vi "Tesla_Test_v3.vi"() -> ()   [LabVIEW 2013]
uses:
  General VIs/Tesla/Control/Command Enum.ctl
  <vilib>/Utility/NIReport.llb/NI_report.lvclass
  <vilib>/Utility/NIReport.llb/Append Report Text (str wrap).vi
  <vilib>/regexp/Match Regular Expression.xnode
panel:
  out "index":i32
  in  "error in":errorcluster
  out "error out":errorcluster
  in  "Tab Control":T1(tab)
  in  "Protocol":bool
  in  "Text Base":bool
  in  "Network":bool
  in  "Commence":bool
  out "IP address":i32
  out "offset past match":i32
  out "concatenated string":string
  out "Ping Cout":i32
  in  "file path":path=path "C:/Users/barddya/Desktop/Tesla/List_of_IPs.txt"
  out "VP/F1 5":bool
  out "VP/F1 4":bool
  out "VP/F1 3":bool
  out "VP/F1 2":bool
  out "VP/F1":bool
  out "Hex 5":bool
  out "Hex 4":bool
  out "Hex 3":bool
  out "Hex 2":bool
  out "Hex 1":bool
  out "Percent 5":dbl
  out "Percent 4":dbl
  out "Percent 3":dbl
  out "Percent 2":dbl
  out "Percent 1":dbl
  out "Voltage 5":dbl
  out "Voltage 4":dbl
  out "Voltage 3":dbl
  out "Voltage 2":dbl
  out "Voltage 1":dbl
  out "Pass/Fail1 5":bool
  out "Pass/Fail1 4":bool
  out "Pass/Fail1 3":bool
  out "Pass/Fail1 2":bool
  out "Pass/Fail1":bool
  in  "Path to Text Base Comm":path=path "C:/Users/barddya/Desktop/Tesla/test2.txt"
  out "Value in Flpating Point":dbl
  out "Hex String":string
  in  "Path Protocol test":path=path "C:/Users/barddya/Desktop/Tesla_Program/test3.bin"
  in  "Panic Stop Stop":bool=TRUE
  in  "Done press continue":bool
  # "Pass/Fail"
  # "Voltage"
  # "Precent"
  # "Is Hex"
  # "Results"
  # "Response 1"
  # "Response 2"
  # "Response 3"
  # "Response 4"
  # "Response 5"
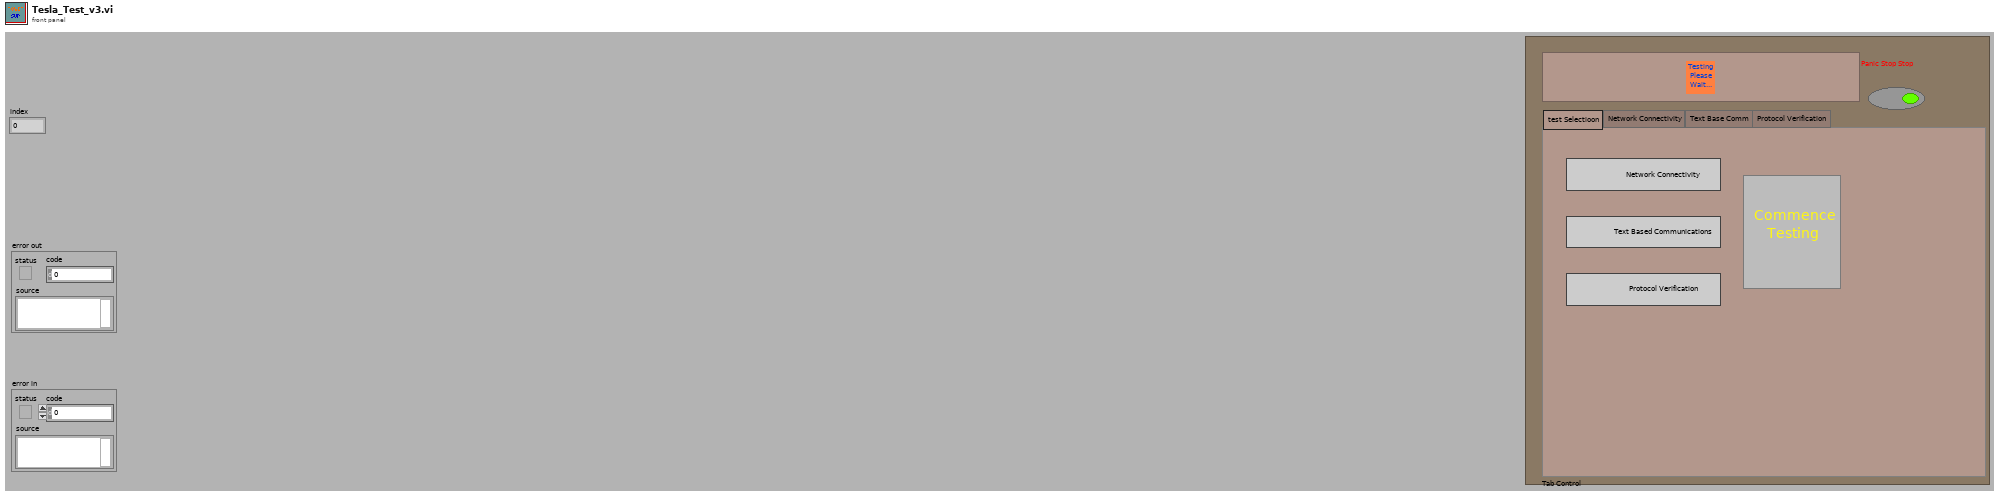
[diagram p1: front panel]
types:
  T1 = enum32{"test Selectioon", "Network Connectivity", "Text Base Comm", "Protocol Verification"}
  T2 = typedef "Command Enum.ctl" = enum16{"Test Selection", "Network", "Text Base", "Protocol", "Restart_Print", "Stop"}
  T3 = enum16{"big-endian, network order", "native, host order", "little-endian"}
  T4 = enum16{"open", "replace", "create", "open or create", "replace or create", "replace or create with confirmation"}
  T5 = cluster{"Charset (-1)":i16, "Weight (-1)":i16, "Name":string, "Size":string}
  T6 = enum16{"Standard Report", "HTML", "Word", "Excel"}
  T7 = cluster{"output state":bool, "Device ID":i32, "Set CC current":dbl}
  T8 = enum16{"Left Button", "Center Button", "Right Button", "Window Close"}
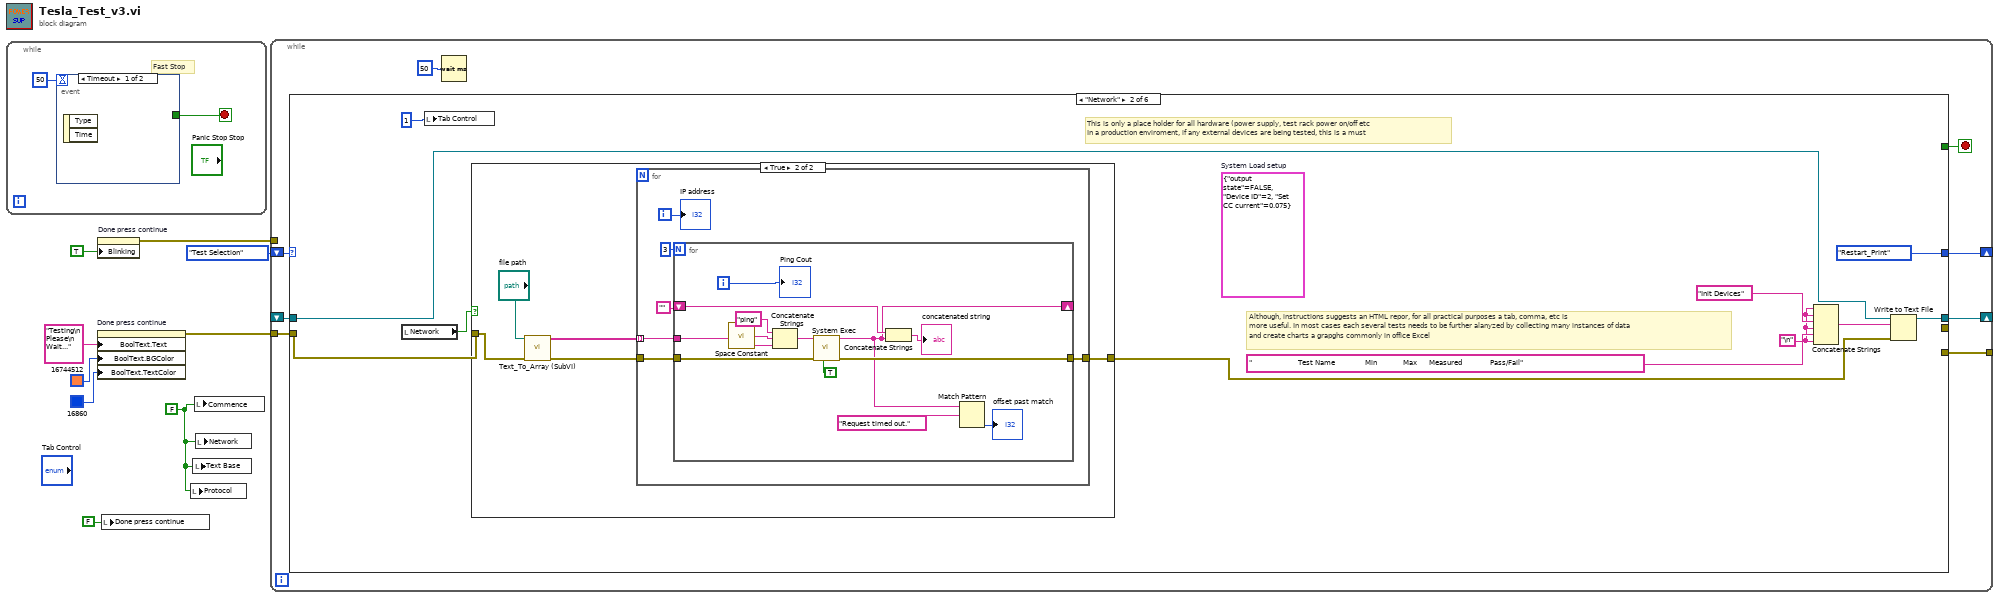
[diagram p0: block diagram]
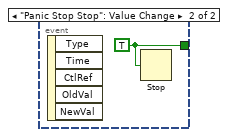
[diagram p2: hidden frame]
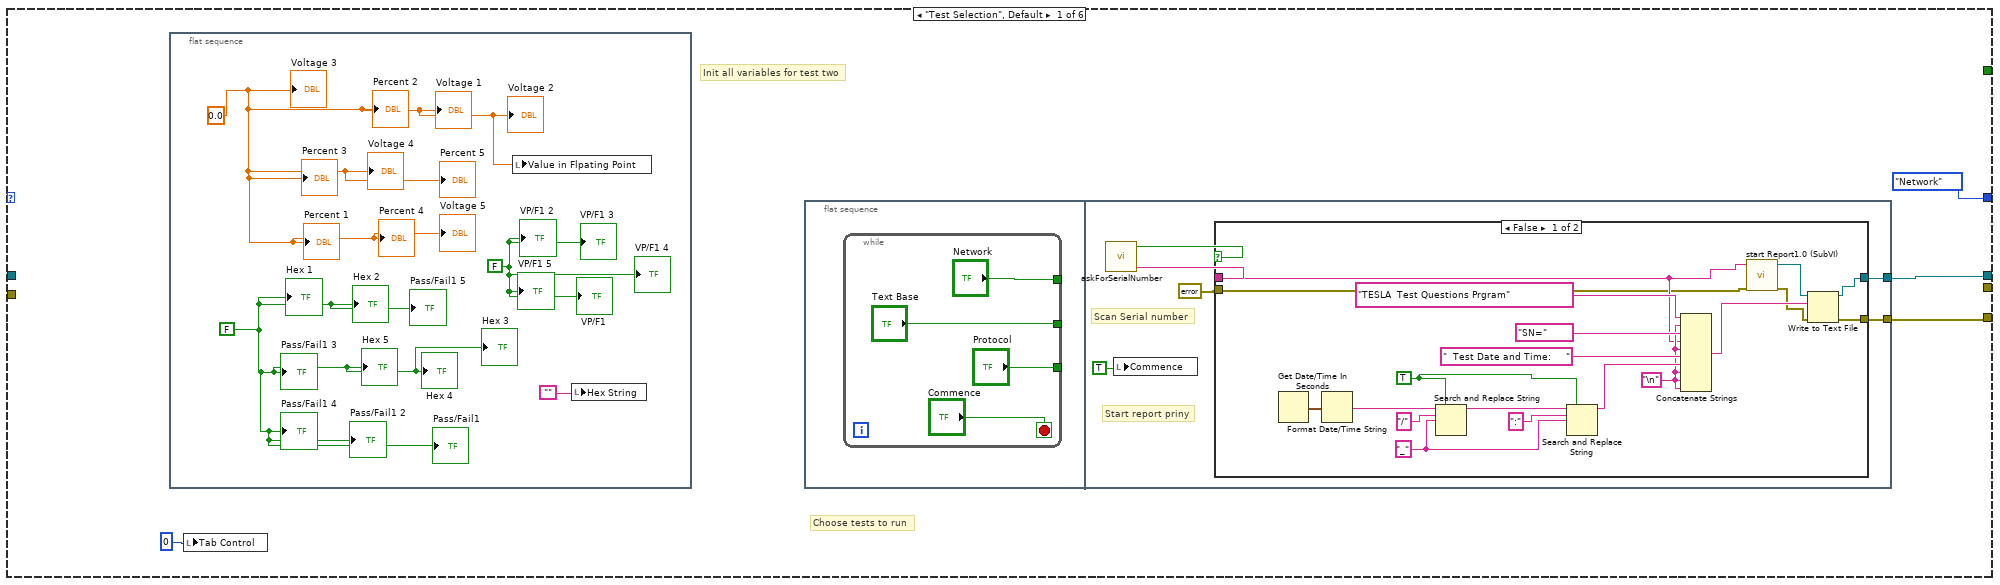
[diagram p3: hidden frame]
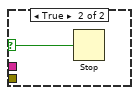
[diagram p4: hidden frame]
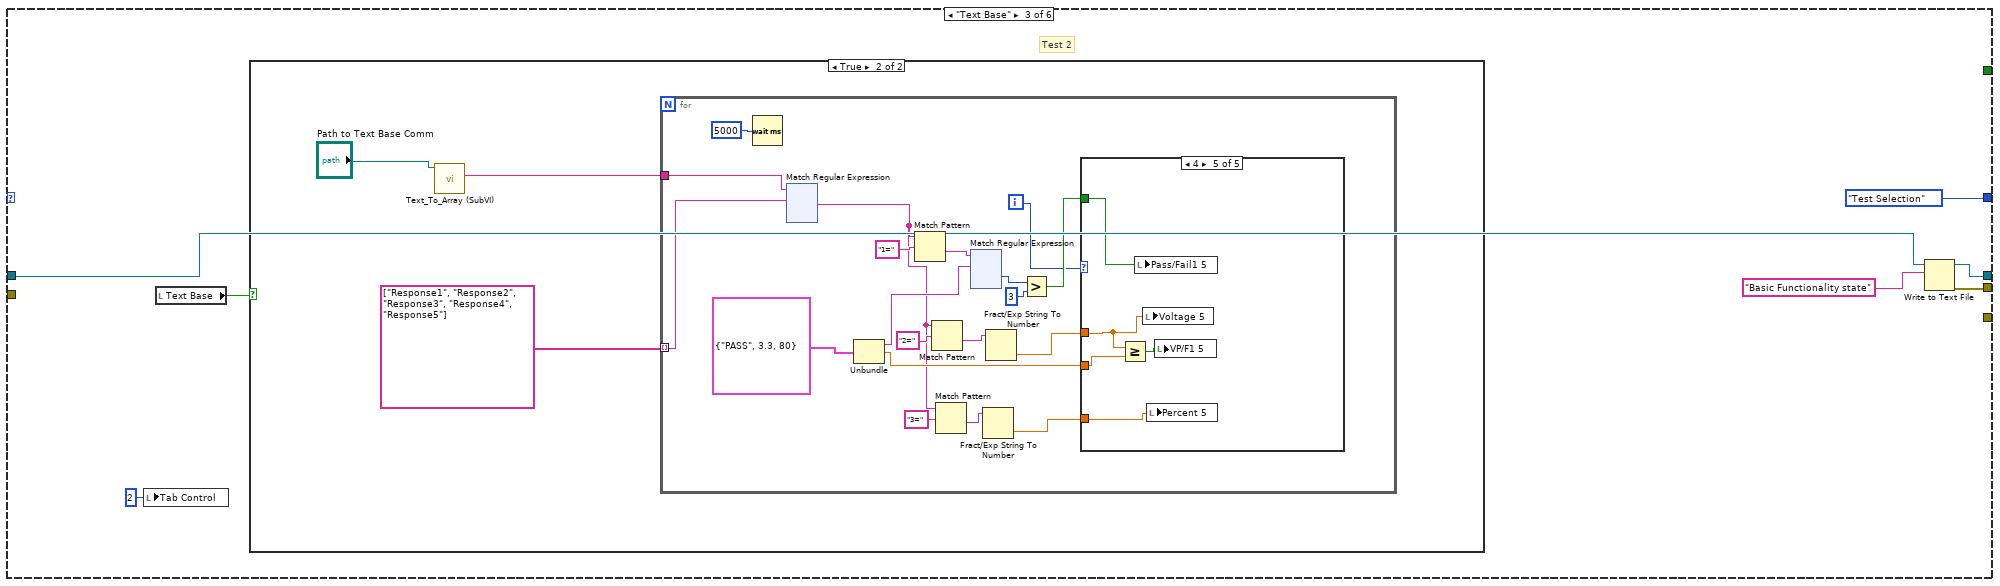
[diagram p6: hidden frame]
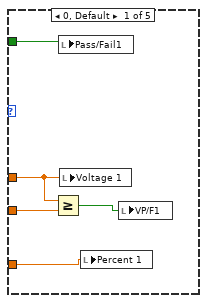
[diagram p8: hidden frame]
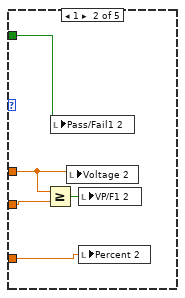
[diagram p9: hidden frame]
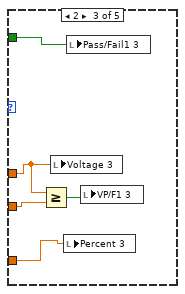
[diagram p10: hidden frame]
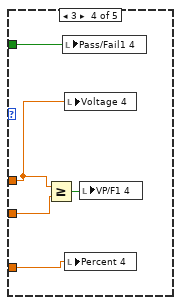
[diagram p11: hidden frame]
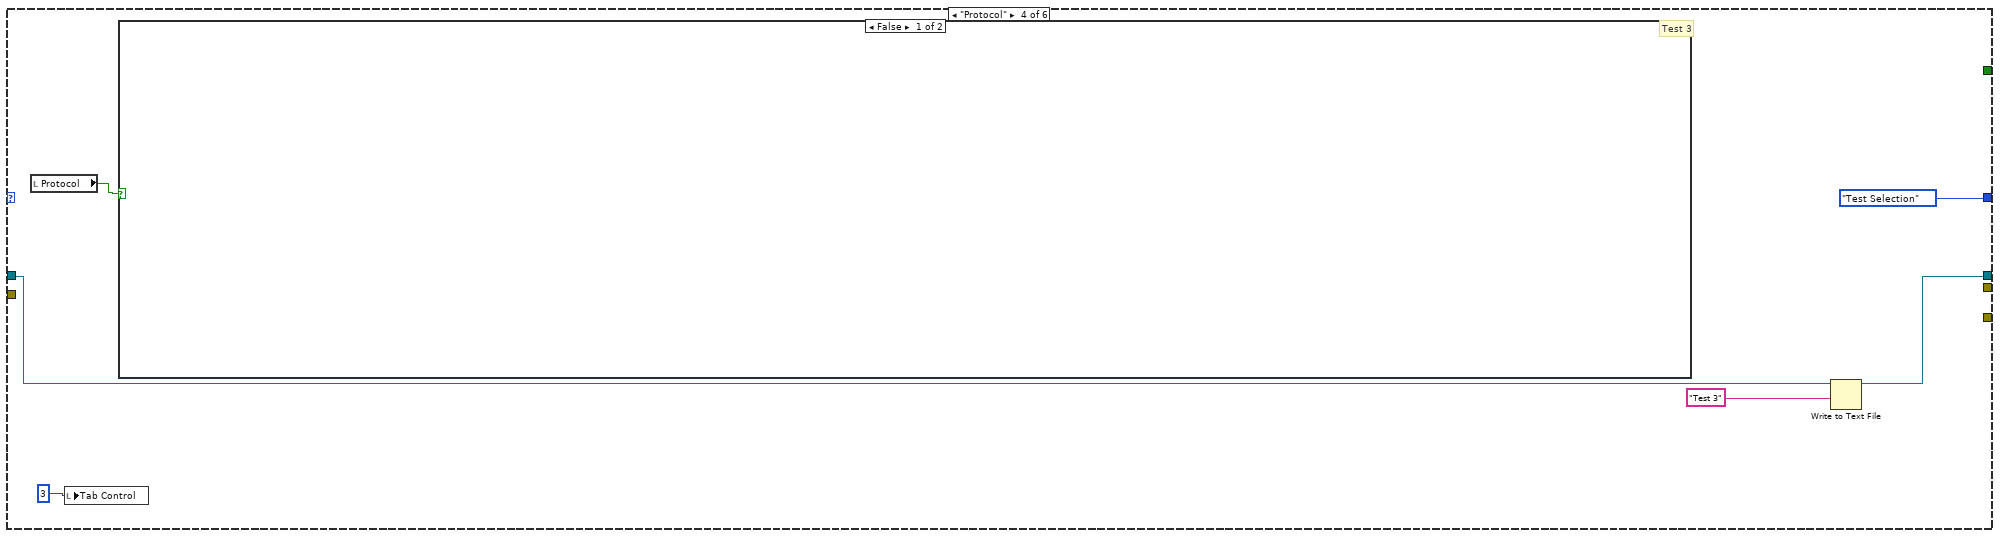
[diagram p12: hidden frame]
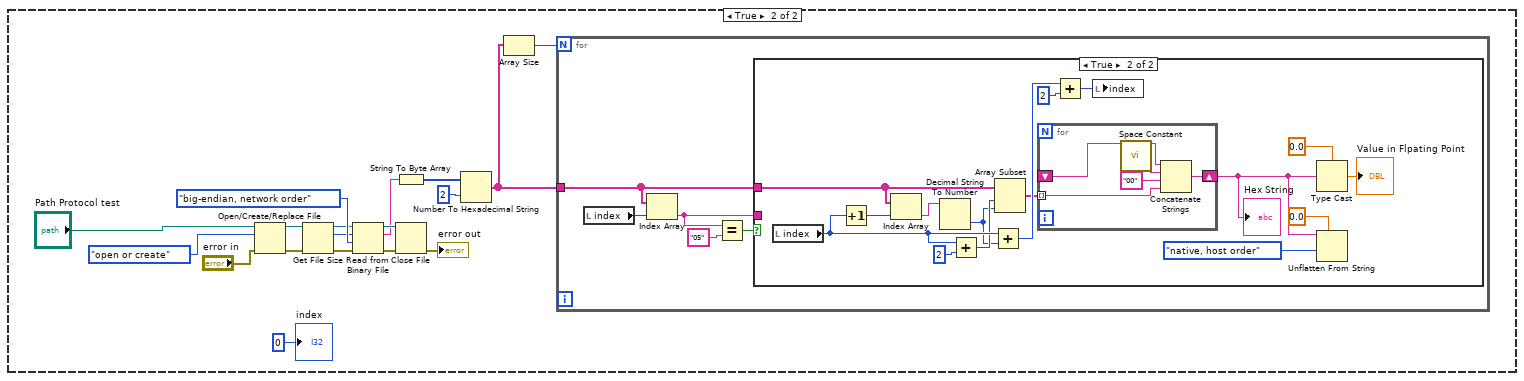
[diagram p13: hidden frame]
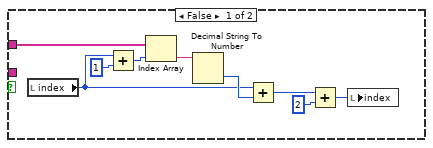
[diagram p14: hidden frame]
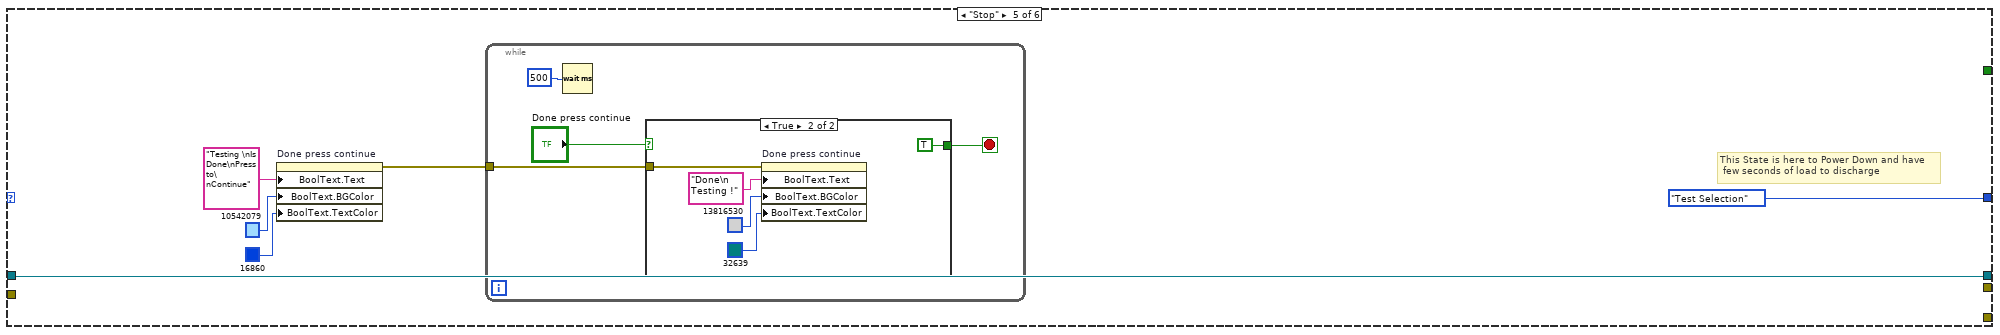
[diagram p15: hidden frame]
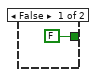
[diagram p16: hidden frame]
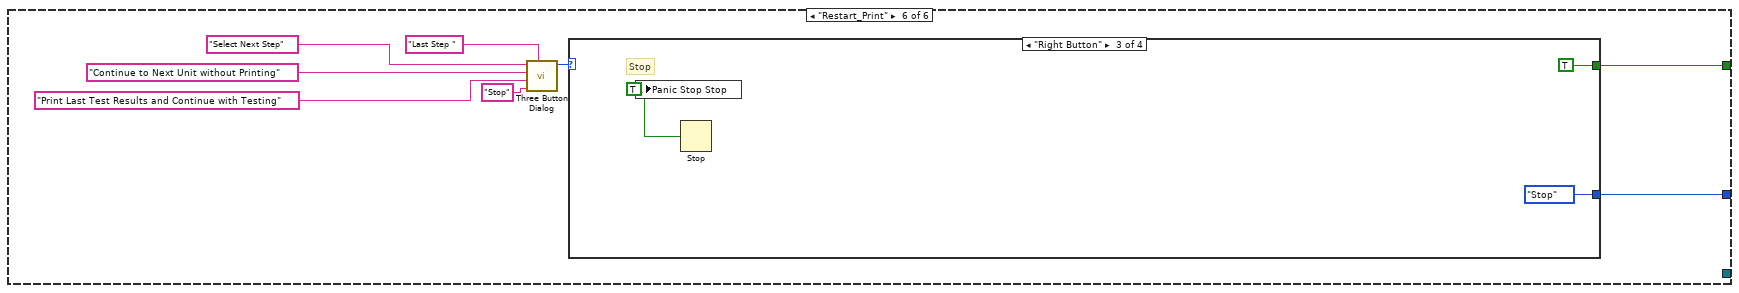
[diagram p17: hidden frame]
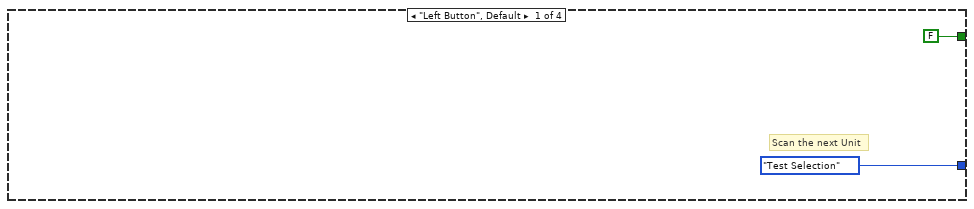
[diagram p18: hidden frame]
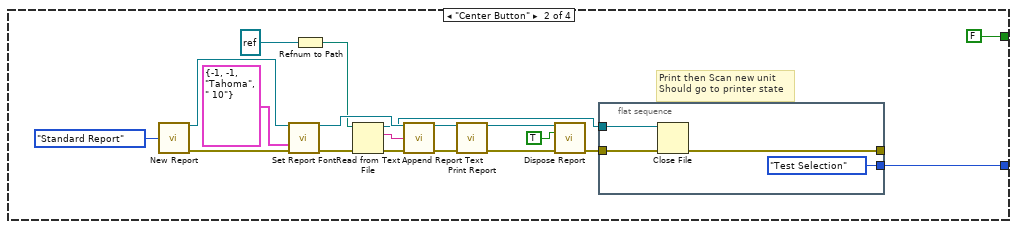
[diagram p19: hidden frame]
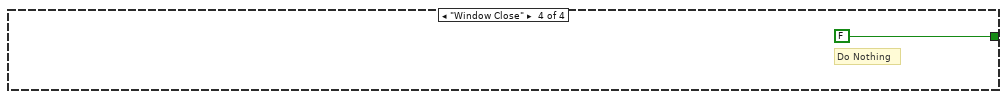
[diagram p20: hidden frame]
diagram:
  w1 = FALSE
  n1 = while {
    stop <- w10 stop-if-true
    # "Fast Stop"
    n2 = event shown="[0] Timeout" {
      selector: _ -> [_ _]
      dyn-events: _ -> [_ _]
      timeout: 50 -> [_ _]
      tunnel: [_ w12] -> w10
      event Timeout {
        n3 = event-data() -> ()  [unwired: 1 in, 2 out]
      }
      event "Panic Stop Stop": Value Change {
        w12 = TRUE
        n4 = event-data() -> ()  [unwired: 1 in, 5 out]
        n5 = Stop(stop? (T)=w12) -> ()
      }
    }
  }
  n6 = property on="Done press continue" class="Bool (strict)"("BoolText.Text"="Testing\n Please\n Wait...", "BoolText.BGColor"=u32 16744512, "BoolText.TextColor"=u32 16860) -> (error out=w7:errorcluster)  [unwired: 2 in, 1 out]
  n7 = property on="Done press continue" class="Bool (strict)"("Blinking"=TRUE) -> (error out=w3:errorcluster)  [unwired: 2 in, 1 out]
  n8 = local write "Done press continue"(FALSE) -> ()
  n9 = local write "Protocol"(w1) -> ()
  n10 = local write "Text Base"(w1) -> ()
  n11 = local write "Commence"(w1) -> ()
  n12 = local write "Network"(w1) -> ()
  n13 = while {
    shift-right: [w19] -> _
    shift-left: Command_Enum."Test Selection" ("Command Enum") -> [w20]
    tunnel: w7 -> [w16]
    tunnel: w3 -> [_]
    shift-right: [w15] -> _
    shift-left: _ -> [w14]
    tunnel: [w13] -> _
    stop <- w18 stop-if-true
    n14 = case shown="\"Network\"" w20 {
      tunnel: [Command_Enum."Network" ("Command Enum") Command_Enum."Restart_Print" ("Command Enum") Command_Enum."Test Selection" ("Command Enum") Command_Enum."Test Selection" ("Command Enum") Command_Enum."Test Selection" ("Command Enum") w453] -> w19
      tunnel: [_ _ _ _ _ w452] -> w18
      tunnel: w16 -> [_ w62 _ _ _ _]
      tunnel: [w23 w67 w99 w381 w436 _] -> w15
      tunnel: w14 -> [_ w66 w98 w379 w436 _]
      tunnel: [_ _ w100 _ _ _] -> _
      tunnel: [w21 _ _ _ _ _] -> w13
      frame "Test Selection", Default {
        # "Choose tests to run"
        # "Init all variables for test two"
        n15 = flat-sequence {
          frame #0 {
            w27 = FALSE
            w28 = FALSE
            w26 = 0.0
            n16 = local write "Value in Flpating Point"(w26) -> ()
            n17 = local write "Hex String"("") -> ()
            "Voltage 5" <- w26
            "Percent 5" <- w26
            "Voltage 3" <- w26
            "Voltage 4" <- w26
            "Voltage 2" <- w26
            "Percent 4" <- w26
            "Percent 3" <- w26
            "Voltage 1" <- w26
            "Percent 2" <- w26
            "Percent 1" <- w26
            "Pass/Fail1 5" <- w28
            "Hex 5" <- w28
            "Pass/Fail1 3" <- w28
            "Pass/Fail1 4" <- w28
            "Pass/Fail1" <- w28
            "Hex 3" <- w28
            "Hex 4" <- w28
            "Hex 2" <- w28
            "Hex 1" <- w28
            "Pass/Fail1 2" <- w28
            "VP/F1 3" <- w27
            "VP/F1 4" <- w27
            "VP/F1 2" <- w27
            "VP/F1" <- w27
            "VP/F1 5" <- w27
          }
        }
        n18 = local write "Tab Control"(0) -> ()
        n19 = flat-sequence {
          tunnel: [w36] -> w23
          tunnel: [w35] -> w21
          frame #0 {
            n20 = while {
              tunnel: ["Network"] -> _
              tunnel: ["Text Base"] -> _
              tunnel: ["Protocol"] -> _
              stop <- "Commence" stop-if-true
            }
          }
          frame #1 {
            # "Start report priny"
            # "Scan Serial number"
            n21 = call "askForSerialNumber.vi"() -> ("Stop"=w38:bool, "Serial Number scanned"=w37:string)  [unwired: 1 in, 1 out]
            n22 = local write "Commence"(TRUE) -> ()
            n23 = case shown="False" w38 {
              selector: w38 -> [_ w58]
              tunnel: w37 -> [w42 _]
              tunnel: [w45 _] -> w36
              tunnel: [w43 _] -> w35
              tunnel: errorcluster {"status"=FALSE, "code"=0, "source"=""} ("error constant") -> [w41 _]
              frame False {
                w46 = "\n"
                w55 = TRUE ("replace all? (F)")
                w54 = "_"
                n24 = Get Date/Time In Seconds() -> (seconds since 1Jan1904=w49:timestamp)
                n25 = Format Date/Time String(seconds (now)=w49) -> (date/time string=w50:string)  [unwired: 2 in]
                n26 = Search and Replace String(replace all?=w55, input string=w50, search string="/", replace string=w54) -> (result string=w52:string)  [unwired: 4 in, 3 out]
                n27 = Search and Replace String(replace all?=w55, input string=w52, search string=":", replace string=w54) -> (result string=w57:string)  [unwired: 4 in, 3 out]
                n28 = Concatenate Strings("TESLA  Test Questions Prgram", w46, "SN=", w42, w46, "  Test Date and Time:     ", w57, w46, w46, w46) -> (w44:string)
                n29 = call "start Report1.0 (SubVI).vi"("error in (no error)"=w41, "Serial Number"=w42) -> ("error out"=w40:errorcluster, "Byte Stream File out"=w39:refnum<file>)  [unwired: 8 in]
                n30 = Write to Text File(file (use dialog)=w39, text=w44, error in=w40) -> (refnum out=w45:refnum<file>, error out=w43:errorcluster)  [unwired: 1 in, 1 out]
              }
              frame True {
                n31 = Stop(stop? (T)=w58) -> ()
              }
            }
          }
        }
      }
      frame "Network" {
        w63 = "\n"
        (unwired) T7 {"output state"=FALSE, "Device ID"=2, "Set CC current"=0.075}  # System Load setup
        # "Although, instructions suggests an HTML repor, for all practical purposes a tab, comma, etc is \nmore useful. In most cases each several tests needs to be further alanyzed by collecting many instances of data \nand create charts a grapghs commonly in office Excel"
        # "This is only a place holder for all hardware (power supply, test rack power on/off etc\nIn a production enviroment, if any external devices are being tested, this is a must"
        n32 = local read "Network"() -> (w59:bool)
        n33 = local write "Tab Control"(1) -> ()
        n34 = case shown="True" w59 {
          tunnel: w62 -> [w70 w72]
          tunnel: [w70 w71] -> w61
          frame False {
          }
          frame True {
            n35 = call "Text_To_Array (SubVI).vi"("error in (no error)"=w72, "file path"="file path") -> ("error out"=w74:errorcluster, "Array"=w75:string[])  [unwired: 7 in, 1 out]
            n36 = for {
              tunnel: w75 -> [w79] mode=indexing
              tunnel: w74 -> [w81]
              tunnel: [w80] -> w71
              i -> [w77]
              n37 = for {
                N: 3 -> [_]
                tunnel: w81 -> [w94]
                tunnel: [w93] -> w80
                tunnel: w79 -> [w91]
                shift-right: [w84] -> _
                shift-left: "" -> [w86]
                i -> [w87]
                n38 = call <vilib>:"Space Constant.vi"() -> ("String"=w89:string)
                n39 = Concatenate Strings("ping", w89, w91) -> (w92:string)
                n40 = call <vilib>:"System Exec.vi"("run minimized? (F)"=TRUE, "error in (no error)"=w94, "command line"=w92) -> ("error out"=w93:errorcluster, "standard output"=w84:string)  [unwired: 5 in, 2 out]
                n41 = Concatenate Strings(w86, w84) -> (→"concatenated string":string)
                n42 = Match Pattern(string=w84, regular expression="Request timed out." ("search string/char (-)")) -> (offset past match=→"offset past match":i32)  [unwired: 1 in, 3 out]
                "Ping Cout" <- w87
              }
              "IP address" <- w77
            }
          }
        }
        n43 = Concatenate Strings(w63, w63, "Init Devices", w63, "                       Test Name               Min             Max      Measured              Pass/Fail", w63) -> (w68:string)
        n44 = Write to Text File(file (use dialog)=w66, text=w68, error in=w61) -> (refnum out=w67:refnum<file>)  [unwired: 1 in, 2 out]
      }
      frame "Text Base" {
        # "Test 2"
        n45 = local write "Tab Control"(2) -> ()
        n46 = local read "Text Base"() -> (w96:bool)
        n47 = case shown="True" w96 {
          frame False {
          }
          frame True {
            n48 = call "Text_To_Array (SubVI).vi"("file path"="Path to Text Base Comm") -> ("text"=w103:string)  [unwired: 8 in, 2 out]
            n49 = for {
              tunnel: w103 -> [w112]
              tunnel: string[] ["Response1", "Response2", "Response3", "Response4", "Response5"] -> [w111] mode=indexing
              i -> [w110]
              n50 = Wait (ms)(milliseconds to wait=5000) -> ()  [unwired: 1 out]
              n51 = xnode "Match Regular Expression"("input string"=w112, "regular expression"=w111) -> ("after match"=w107:string)  [unwired: 4 in, 4 out]
              n52 = Unbundle(cluster{string, dbl, i32} {"PASS", 3.3, 80}) -> (w122:string, w109:dbl)  [unwired: 1 out]
              n53 = Match Pattern(string=w107, regular expression="1=") -> (after substring=w119:string)  [unwired: 1 in, 3 out]
              n54 = Match Pattern(string=w107, regular expression="2=") -> (after substring=w114:string)  [unwired: 1 in, 3 out]
              n55 = Match Pattern(string=w107, regular expression="3=") -> (after substring=w106:string)  [unwired: 1 in, 3 out]
              n56 = xnode "Match Regular Expression"("input string"=w119, "regular expression"=w122) -> ("offset past match"=w118:i32)  [unwired: 4 in, 4 out]
              n57 = Fract/Exp String To Number(string=w106) -> (number=w105:dbl)  [unwired: 3 in, 1 out]
              n58 = Fract/Exp String To Number(string=w114) -> (number=w113:dbl)  [unwired: 3 in, 1 out]
              n59 = Greater?(x=w118, y=3) -> (0:w116:bool)
              n60 = case shown="4" w110 {
                tunnel: w116 -> [w128 w133 w138 w143 w148]
                tunnel: w113 -> [w127 w132 w137 w142 w147]
                tunnel: w109 -> [w126 w131 w136 w141 w146]
                tunnel: w105 -> [w124 w129 w134 w139 w144]
                frame 0, Default {
                  n61 = Greater Or Equal?(x=w127, y=w126) -> (x >= y?=w125:bool)
                  n62 = local write "Pass/Fail1"(w128) -> ()
                  n63 = local write "Voltage 1"(w127) -> ()
                  n64 = local write "Percent 1"(w124) -> ()
                  n65 = local write "VP/F1"(w125) -> ()
                }
                frame 1 {
                  n66 = Greater Or Equal?(x=w132, y=w131) -> (x >= y?=w130:bool)
                  n67 = local write "Pass/Fail1 2"(w133) -> ()
                  n68 = local write "Voltage 2"(w132) -> ()
                  n69 = local write "VP/F1 2"(w130) -> ()
                  n70 = local write "Percent 2"(w129) -> ()
                }
                frame 2 {
                  n71 = Greater Or Equal?(x=w137, y=w136) -> (x >= y?=w135:bool)
                  n72 = local write "Voltage 3"(w137) -> ()
                  n73 = local write "Percent 3"(w134) -> ()
                  n74 = local write "Pass/Fail1 3"(w138) -> ()
                  n75 = local write "VP/F1 3"(w135) -> ()
                }
                frame 3 {
                  n76 = Greater Or Equal?(x=w142, y=w141) -> (x >= y?=w140:bool)
                  n77 = local write "Pass/Fail1 4"(w143) -> ()
                  n78 = local write "Voltage 4"(w142) -> ()
                  n79 = local write "Percent 4"(w139) -> ()
                  n80 = local write "VP/F1 4"(w140) -> ()
                }
                frame 4 {
                  n81 = Greater Or Equal?(x=w147, y=w146) -> (x >= y?=w145:bool)
                  n82 = local write "Pass/Fail1 5"(w148) -> ()
                  n83 = local write "Voltage 5"(w147) -> ()
                  n84 = local write "Percent 5"(w144) -> ()
                  n85 = local write "VP/F1 5"(w145) -> ()
                }
              }
            }
          }
        }
        n86 = Write to Text File(file (use dialog)=w98, text="Basic Functionality state") -> (refnum out=w99:refnum<file>, error out=w100:errorcluster)  [unwired: 2 in, 1 out]
      }
      frame "Protocol" {
        # "Test 3"
        n87 = local read "Protocol"() -> (w378:bool)
        n88 = local write "Tab Control"(3) -> ()
        n89 = case shown="False" w378 {
          frame False {
          }
          frame True {
            n90 = Open/Create/Replace File(file path (use dialog)="Path Protocol test", error in="error in", operation (0:open)=T4."open or create") -> (refnum out=w393:refnum<file>, error out=w391:errorcluster)  [unwired: 3 in, 1 out]
            n91 = Get File Size(file=w393, error in=w391) -> (refnum out=w392:refnum<file>, size (in bytes)=w389:i64, 0:w390:errorcluster)
            n92 = Read from Binary File(8:w390, 9:T3."big-endian, network order" ("byte order (0:big-endian, network order)"), 10:w389, 11:w392) -> (0:w396:errorcluster, 2:w388:string, 3:w394:refnum<file>)  [unwired: 2 in, 1 out]
            n93 = String To Byte Array(string=w388) -> (unsigned byte array=w387:u8[])
            n94 = Close File(refnum=w394, error in=w396) -> (error out=→"error out":errorcluster)  [unwired: 1 out]
            n95 = Number To Hexadecimal String(1:2, 2:w387) -> (0:w385:string[])
            n96 = Array Size(array=w385) -> (size(s)=w383:i32)
            n97 = for {
              N: w383 -> [_]
              tunnel: w385 -> [w403]
              n98 = local read "index"() -> (w401:i32)
              n99 = Index Array(array=w403, index=w401) -> (element=w402:string)
              n100 = Equal?(x=w402, y="05") -> (x = y?=w404:bool)
              n101 = case shown="True" w404 {
                tunnel: w403 -> [w412 w427]
                tunnel: w402 -> [_ _]
                frame False {
                  n102 = local read "index"() -> (w409:i32)
                  n103 = Add(x=w409, y=1) -> (x+y=w410:i32)
                  n104 = Index Array(array=w412, index=w410) -> (element=w414:string)
                  n105 = Decimal String To Number(string=w414) -> (number=w413:i32)  [unwired: 2 in, 1 out]
                  n106 = Add(x=w409, y=w413) -> (x+y=w408:i32)
                  n107 = Add(x=w408, y=2) -> (x+y=w406:i32)
                  n108 = local write "index"(w406) -> ()
                }
                frame True {
                  n109 = local read "index"() -> (w425:i32)
                  n110 = Increment(x=w425) -> (x+1=w430:i32)
                  n111 = Index Array(array=w427, index=w430) -> (element=w428:string)
                  n112 = Decimal String To Number(string=w428) -> (number=w421:i32)  [unwired: 2 in, 1 out]
                  n113 = Add(x=w425, y=2) -> (x+y=w423:i32)
                  n114 = Add(x=w425, y=w421) -> (x+y=w426:i32)
                  n115 = Array Subset(array=w427, index=w423, length=w421) -> (w420:string[])
                  n116 = for {
                    tunnel: w420 -> [w434] mode=indexing
                    shift-right: [w435] -> w416
                    shift-left: _ -> [w433]
                    n117 = call <vilib>:"Space Constant.vi"() -> ("String"=w431:string)
                    n118 = Concatenate Strings(w433, w431, "00", w434) -> (w435:string)
                  }
                  "Hex String" <- w416
                  n119 = Add(x=w426, y=2) -> (x+y=w422:i32)
                  n120 = local write "index"(w422) -> ()
                  n121 = Type Cast(type=0.0, x=w416) -> (*(type *) &x=→"Value in Flpating Point":dbl)
                  n122 = Unflatten From String(type=0.0, binary string=w416, byte order (0:big-endian, network order)=T3."native, host order") -> ()  [unwired: 2 in, 3 out]
                }
              }
            }
            "index" <- 0
          }
        }
        n123 = Write to Text File(file (use dialog)=w379, text="Test 3") -> (refnum out=w381:refnum<file>)  [unwired: 2 in, 2 out]
      }
      frame "Stop" {
        # "This State is here to Power Down and have\n few seconds of load to discharge"
        n124 = property on="Done press continue" class="Bool (strict)"("BoolText.Text"="Testing \nIs Done\nPress to\nContinue", "BoolText.BGColor"=u32 10542079, "BoolText.TextColor"=u32 16860) -> (error out=w440:errorcluster)  [unwired: 2 in, 1 out]
        n125 = while {
          tunnel: w440 -> [w443]
          stop <- w442 stop-if-true
          n126 = Wait (ms)(milliseconds to wait=500) -> ()  [unwired: 1 out]
          n127 = case shown="True" "Done press continue" {
            tunnel: [FALSE TRUE] -> w442
            tunnel: w443 -> [_ w448]
            frame False {
            }
            frame True {
              n128 = property on="Done press continue" class="Bool (strict)"(error in=w448, "BoolText.Text"="Done\n Testing !", "BoolText.BGColor"=u32 13816530, "BoolText.TextColor"=u32 32639) -> ()  [unwired: 1 in, 2 out]
            }
          }
        }
      }
      frame "Restart_Print" {
        n129 = call <vilib>:"Three Button Dialog.vi"("Window Title (\"\")"="Last Step " ("Window Title (\"\")"), "Right Button Text (\"Cancel\")"="Stop" ("Window Title (\"\")"), "Center Button Text (\"No\")"="Print Last Test Results and Continue with Testing" ("Window Title (\"\")"), "Left Button Text (\"Yes\")"="Continue to Next Unit without Printing" ("Window Title (\"\")"), "message"="Select Next Step" ("Window Title (\"\")")) -> ("Which Button?"=w459:T8)  [unwired: 6 in]
        n130 = case shown="\"Right Button\"" w459 {
          tunnel: [Command_Enum."Test Selection" ("Command Enum") w464 Command_Enum."Stop" ("Command Enum") _] -> w453
          tunnel: [FALSE FALSE TRUE FALSE] -> w452
          frame "Left Button", Default {
            # "Scan the next Unit"
          }
          frame "Center Button" {
            # "Print then Scan new unit\nShould go to printer state"
            n131 = call <vilib>:"New Report.vi"("report type"=T6."Standard Report") -> ("report out"=w477:refnum<class "NI_report.lvclass">, "error out"=w478:errorcluster)  [unwired: 13 in]
            n132 = call-dynamic "Set Report Font.vi"("report in"=w477, "font settings"=T5 {"Charset (-1)"=-1, "Weight (-1)"=-1, "Name"="Tahoma", "Size"=" 10"}, "error in (no error)"=w478) -> ("report out"=w476:refnum<class "NI_report.lvclass">, "error out"=w475:errorcluster)  [unwired: 10 in, 1 out]
            n133 = Refnum to Path(1:refnum<file> refnum ("refnum")) -> (0:w463:path)
            n134 = Read from Text File(file (use dialog)=w463, error in=w475) -> (refnum out=w465:refnum<file>, text=w474:string, error out=w473:errorcluster)  [unwired: 2 in, 1 out]
            n135 = call-poly <vilib>:"Append Report Text.vi"("report in"=w476, "text"=w474, "error in (no error)"=w473) -> ("report out"=w472:refnum<class "NI_report.lvclass">, "error out"=w469:errorcluster)  [unwired: 9 in, 2 out]
            n136 = call-dynamic "Print Report.vi"("report in"=w472, "error in (no error)"=w469) -> ("report out"=w470:refnum<class "NI_report.lvclass">, "error out"=w471:errorcluster)  [unwired: 12 in]
            n137 = call-dynamic "Dispose Report.vi"("report in"=w470, "wait until printing completed? (T)"=TRUE, "error in (no error)"=w471) -> ("error out"=w466:errorcluster)  [unwired: 12 in]
            n138 = flat-sequence {
              tunnel: w466 -> [w484]
              tunnel: [w483] -> _
              tunnel: w465 -> [w482]
              tunnel: [Command_Enum."Test Selection" ("Command Enum")] -> w464
              frame #0 {
                n139 = Close File(refnum=w482, error in=w484) -> (error out=w483:errorcluster)  [unwired: 1 out]
              }
            }
          }
          frame "Right Button" {
            w485 = TRUE
            # "Stop"
            n140 = local write "Panic Stop Stop"(w485) -> ()
            n141 = Stop(stop? (T)=w485) -> ()
          }
          frame "Window Close" {
            # "Do Nothing"
          }
        }
      }
    }
    n142 = Wait (ms)(milliseconds to wait=50) -> ()  [unwired: 1 out]
  }
